vi "Result_Test.vi"(8 "error in (no error)":errorcluster caption="entrée d'erreur (pas d'erreur)", 11 "Get_Voltage en entrée":refnum<class "Zigbee_Stop_Permit_Join.lvclass">) -> (0 "error out":errorcluster caption="sortie d'erreur", 3 "Get_Voltage en sortie":refnum<class "Zigbee_Stop_Permit_Join.lvclass">)   [LabVIEW 2020, in "Library Test.lvlib" / "Zigbee_Stop_Permit_Join.lvclass"]
uses:
  Zigbee_Stop_Permit_Join.lvclass
  C:/Users/ngarcin/OneDrive - Altyor/Standard TB/Class/Test/Test (Default)/Test (Default).lvclass
  Zigbee_Send_Command_UART/Zigbee_Send_Command_UART.lvclass
  Zigbee_Stop_Permit_Join.lvclass/Zigbee_Stop_Permit_Join.ctl
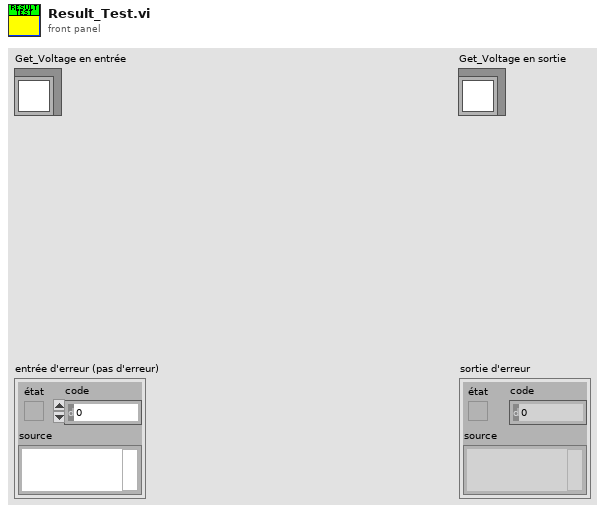
[diagram p1: front panel]
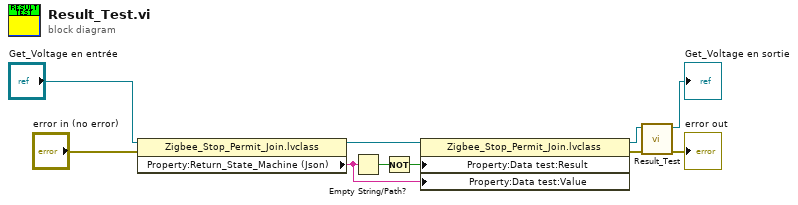
[diagram p0: block diagram]
diagram:
  n1 = property class="Zigbee_Stop_Permit_Join.lvclass"(reference="Get_Voltage en entrée", error in="error in (no error)") -> (reference out=w8:refnum<class "Zigbee_Stop_Permit_Join.lvclass">, "Property:Return_State_Machine (Json)"=w1:string)  [unwired: 1 out]
  n2 = Empty String/Path?(string/path=w1) -> (empty?=w3:bool)
  n3 = Not(x=w3) -> (.not. x?=w2:bool)
  n4 = property class="Zigbee_Stop_Permit_Join.lvclass"(reference=w8, "Property:Data test:Result"=w2, "Property:Data test:Value"=w1) -> (reference out=w5:refnum<class "Zigbee_Stop_Permit_Join.lvclass">, error out=w4:errorcluster)  [unwired: 1 in]
  n5 = call-parent "Result_Test.vi"("error in (no error)"=w4, "Get_Voltage en entrée"=w5) -> ("error out"=→"error out":errorcluster, "Get_Voltage en sortie"=→"Get_Voltage en sortie":refnum<class "Zigbee_Stop_Permit_Join.lvclass">)  [unwired: 8 in]
